vi "Assert Connections.vi"(8 "error in":errorcluster, 10 "actual connections":T1[](array[typedef]), 11 "expected connections":T1[](array[typedef])) -> (0 "error out":errorcluster, 2 "result":string, 3 "pass":bool)   [LabVIEW 2020, in "MeasurementServerTests.lvlib"]
uses:
  MeasurementServerTests.lvlib
  Runtime/MeasurementLink Session Management/Session Reservation/Connection with Session.ctl
  Runtime/MeasurementLink Session Management/Session Reservation/Connection.ctl
  94283ac5-2298-4b3a-b57d-7be67da3787d.vi
  f7d9c9cb-0251-4d67-81cb-70e1b0e8b69f.vi
  <vilib>/JDP Science/JSONtext/Variant to JSON Text.vi
  <vilib>/JDP Science/JSONtext/LVClass Serializer/JSONtext LVClass Serializer.lvclass
  Runtime/MeasurementLink Session Management/Session Reservation/Session Reservation.lvclass
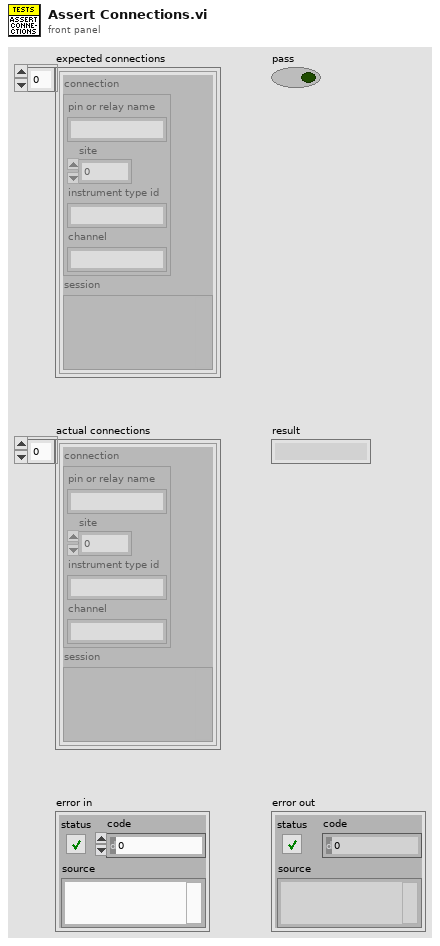
[diagram p1: front panel]
types:
  T1 = typedef "MeasurementLink Session Management.lvlib/Session Reservation.lvclass/Connection with Session.ctl" = cluster{"connection":T2, "session":variant}
  T2 = typedef "MeasurementLink Session Management.lvlib/Session Reservation.lvclass/Connection.ctl" = cluster{"pin or relay name":string, "site":i32, "instrument type id":string, "channel":string}
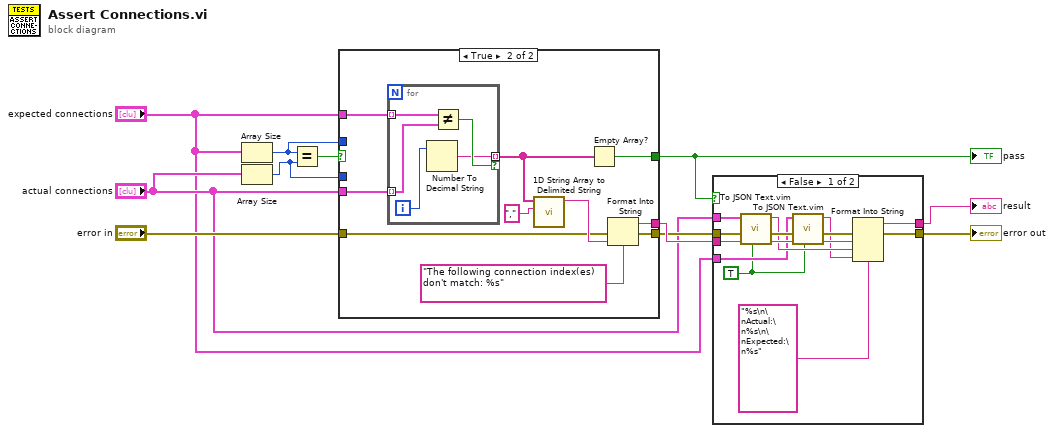
[diagram p0: block diagram]
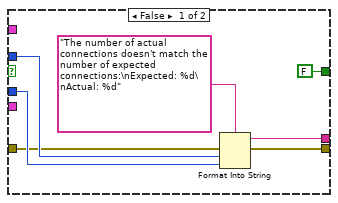
[diagram p3: hidden frame]
diagram:
  n1 = Array Size(array="expected connections") -> (size(s)=w10:i32)
  n2 = Array Size(array="actual connections") -> (size(s)=w11:i32)
  n3 = Equal?(x=w10, y=w11) -> (x = y?=w8:bool)
  n4 = case shown="True" w8 {
    tunnel: "expected connections" -> [_ w28]
    tunnel: "actual connections" -> [_ w27]
    tunnel: [FALSE ("empty?") w22] -> w9
    tunnel: w10 -> [w16 _]
    tunnel: w11 -> [w15 _]
    tunnel: [w17 w21] -> w7
    tunnel: "error in" -> [w14 w20]
    tunnel: [w13 w19] -> w5
    frame False {
      n5 = Format Into String(format string="The number of actual connections doesn't match the number of expected connections:\nExpected: %d\nActual: %d" ("string"), error in=w14, w16, w15) -> (resulting string=w17:string, error out=w13:errorcluster)  [unwired: 1 in]
    }
    frame True {
      n6 = for {
        tunnel: w28 -> [w33] mode=indexing
        tunnel: w27 -> [w32] mode=indexing
        tunnel: [w29] -> w23 mode=indexing if=w30
        i -> [w31]
        n7 = Number To Decimal String(number=w31) -> (decimal integer string=w29:string)  [unwired: 1 in]
        n8 = Not Equal?(x=w33, y=w32) -> (x != y?=w30:bool)
      }
      n9 = call <vilib>:"1D String Array to Delimited String.vi"("delimiter"=",", "string array"=w23) -> ("delimited string"=w24:string)  [unwired: 9 in]
      n10 = Empty Array?(array=w23) -> (empty?=w22:bool)
      n11 = Format Into String(format string="The following connection index(es) don't match: %s" ("string"), error in=w20, w24) -> (resulting string=w21:string, error out=w19:errorcluster)  [unwired: 1 in]
    }
  }
  "pass" <- w9
  n12 = case shown="False" w9 {
    tunnel: [w45 _] -> w3
    tunnel: w7 -> [w43 _]
    tunnel: w5 -> [w42 w46]
    tunnel: [w39 w46] -> w4
    tunnel: "actual connections" -> [w36 _]
    tunnel: "expected connections" -> [w35 _]
    frame False {
      w34 = TRUE ("Pretty Print?")
      n13 = call "To JSON Text.vim"("Pretty Print?"=w34, "error in (no error)"=w42, "Anything"=w36) -> ("error out"=w41:errorcluster, "<JSON>"=w38:string)  [unwired: 7 in]
      n14 = call "To JSON Text.vim"("Pretty Print?"=w34, "error in (no error)"=w41, "Anything"=w35) -> ("error out"=w40:errorcluster, "<JSON>"=w37:string)  [unwired: 7 in]
      n15 = Format Into String(format string="%s\n\nActual:\n%s\n\nExpected:\n%s", error in=w40, w43, w38, w37) -> (resulting string=w45:string, error out=w39:errorcluster)  [unwired: 1 in]
    }
    frame True {
    }
  }
  "error out" <- w4
  "result" <- w3
